vi "FPGA_CounterEncoderSourceConvertionFPGATypeToLVSourceType.vi"(11 "FPGASource":T5={"Channel"=2.0, "Module"=0.0, "AnalogTrigger"=FALSE}) -> (3 "DigitalSource":T1={"DevStatus"={"status"=FALSE, "code"=0, "source"=""}, "AnalogTriggerMode?"=FALSE, "DigitalMode"={"DIO Channel"=enum."DIO 1"}, "AnalogTriggerMode"={"AnalogTriggerIndex"=enum."Trig 0", "OutputType"=enum."InWindow"}})   [LabVIEW 2017]
uses:
  <vilib>/Rock Robotics/SystemInterfaces/CounterEncoderSourceConvertion/FPGA_CounterEncoderSourceConvertionLVSourceType.ctl
  <vilib>/Rock Robotics/SystemInterfaces/DIO/FPGA_DIODigitalSourceChannel.ctl
  <vilib>/Rock Robotics/SystemInterfaces/AnalogTrigger/FPGA_AnalogTriggerIndex.ctl
  <vilib>/Rock Robotics/SystemInterfaces/AnalogTrigger/FPGA_AnalogTriggerOutType.ctl
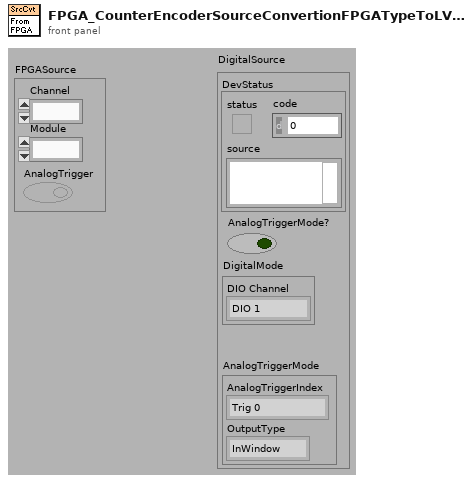
[diagram p1: front panel]
types:
  T1 = typedef "FPGA_CounterEncoderSourceConvertionLVSourceType.ctl" = cluster{"DevStatus":errorcluster, "AnalogTriggerMode?":bool, "DigitalMode":cluster{"DIO Channel":T2}, "AnalogTriggerMode":cluster{"AnalogTriggerIndex":T3, "OutputType":T4}}
  T2 = typedef "FPGA_DIODigitalSourceChannel.ctl" = enum8{"DIO 0", "DIO 1", "DIO 2", "DIO 3", "DIO 4", "DIO 5", "DIO 6", "DIO 7", "DIO 8", "DIO 9", "DIO MXP 0", "DIO MXP 1", "DIO MXP 2", "DIO MXP 3", "DIO MXP 4", "DIO MXP 5", "DIO MXP 6", "DIO MXP 7", "DIO MXP 8", "DIO MXP 9", "DIO MXP 10", "DIO MXP 11", "DIO MXP 12", "DIO MXP 13", "DIO MXP 14", "DIO MXP 15", "Disabled"}
  T3 = typedef "FPGA_AnalogTriggerIndex.ctl" = enum8{"Trig 0", "Trig 1", "Trig 2", "Trig 3", "Trig 4", "Trig 5", "Trig 6", "Trig 7", "Invalid"}
  T4 = typedef "FPGA_AnalogTriggerOutType.ctl" = enum16{"InWindow", "TriggerState", "Rising", "Falling"}
  T5 = cluster{"Channel":fxp<+,4,4>, "Module":fxp<+,1,1>, "AnalogTrigger":bool}
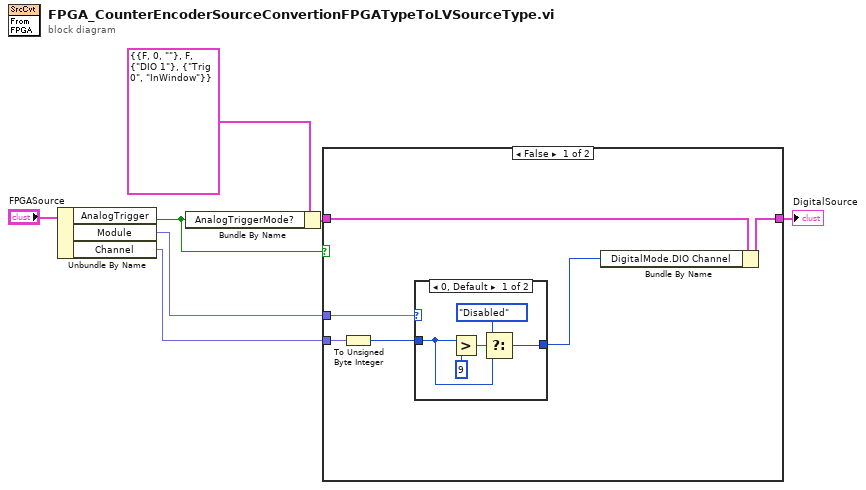
[diagram p0: block diagram]
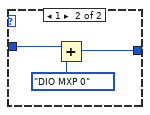
[diagram p2: hidden frame]
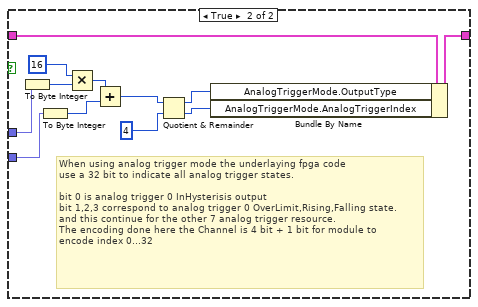
[diagram p3: hidden frame]
diagram:
  n1 = Unbundle By Name("FPGASource") -> ("AnalogTrigger"=w4:bool, "Module"=w3:fxp<+,1,1>, "Channel"=w2:fxp<+,4,4>)
  n2 = Bundle By Name(cluster=T1 {"DevStatus"={"status"=FALSE, "code"=0, "source"=""}, "AnalogTriggerMode?"=FALSE, "DigitalMode"={"DIO Channel"=enum."DIO 1"}, "AnalogTriggerMode"={"AnalogTriggerIndex"=enum."Trig 0", "OutputType"=enum."InWindow"}} ("CounterOrEncoderSource"), "AnalogTriggerMode?"=w4) -> (w5:T1)
  n3 = case shown="False" w4 {
    tunnel: w5 -> [w12 w25]
    tunnel: w3 -> [w10 w31]
    tunnel: w2 -> [w13 w29]
    tunnel: [w11 w24] -> w1
    frame False {
      n4 = To Unsigned Byte Integer(number=w13) -> (unsigned 8bit integer=w9:u8)
      n5 = case shown="0, Default" w10 {
        tunnel: w9 -> [w15 w21]
        tunnel: [w14 w20] -> w8
        frame 0, Default {
          n6 = Greater?(x=w15, y=u8 9) -> (0:w17:bool)
          n7 = Select(t=FPGA_DIODigitalSourceChannel."Disabled" ("DigitalMode.DIO Channel"), s=w17, f=w15) -> (s? t:f=w14:u8)
        }
        frame 1 {
          n8 = Add(x=w21, y=FPGA_DIODigitalSourceChannel."DIO MXP 0" ("DigitalMode.DIO Channel")) -> (x+y=w20:u8)
        }
      }
      n9 = Bundle By Name(cluster=w12, "DigitalMode.DIO Channel"=w8) -> (w11:T1)
    }
    frame True {
      # "When using analog trigger mode the underlaying fpga code\nuse a 32 bit to indicate all analog trigger states.\n\nbit 0 is analog trigger 0 InHysterisis output\nbit 1,2,3 correspond to analog trigger 0 OverLimit,Rising,Falling state.\nand this continue for the other 7 analog trigger resource.\nThe encoding done here the Channel is 4 bit + 1 bit for module to \nencode index 0...32"
      n10 = To Byte Integer(number=w31) -> (8bit integer=w30:i8)
      n11 = To Byte Integer(number=w29) -> (8bit integer=w28:i8)
      n12 = Multiply(x=i8 16, y=w30) -> (x*y=w32:i8)
      n13 = Add(x=w32, y=w28) -> (x+y=w27:i8)
      n14 = Quotient & Remainder(x=w27, y=4) -> (x-y*floor(x/y)=w22:i32, floor(x/y)=w23:i32)
      n15 = Bundle By Name(cluster=w25, "AnalogTriggerMode.OutputType"=w22, "AnalogTriggerMode.AnalogTriggerIndex"=w23) -> (w24:T1)
    }
  }
  "DigitalSource" <- w1
